vi "getDescription.vi"(8 "error in (no error)":errorcluster, 11 "Mocha in":refnum<class "Mocha.lvclass">) -> (0 "error out":errorcluster, 2 "description":string, 3 "Mocha out":refnum<class "Mocha.lvclass">)   [LabVIEW 2017, in "Mocha.lvclass"]
uses:
  Mocha.lvclass
  CondimentDecorator/CondimentDecorator.lvclass
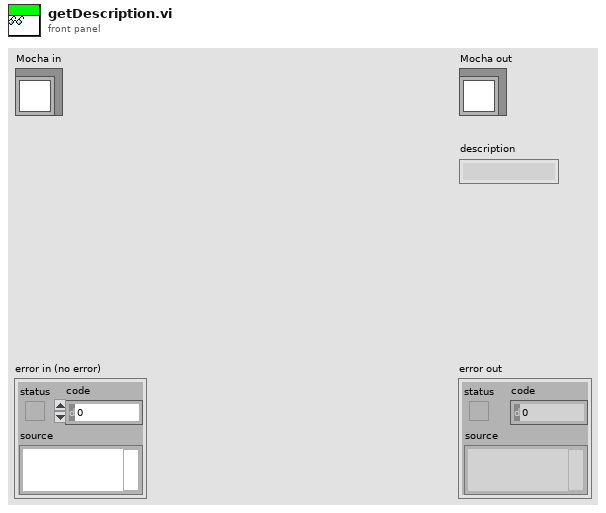
[diagram p1: front panel]
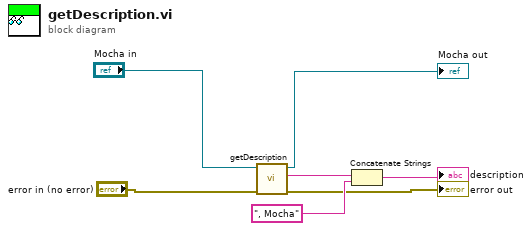
[diagram p0: block diagram]
diagram:
  n1 = call-parent "getDescription.vi"("error in (no error)"="error in (no error)", "CondimentDecorator in"="Mocha in") -> ("error out"=→"error out":errorcluster, "description"=w3:string, "CondimentDecorator out"=→"Mocha out":refnum<class "Mocha.lvclass">)  [unwired: 7 in]
  n2 = Concatenate Strings(w3, ", Mocha") -> (→"description":string)
